vi "Fct_Direction_vent.vi"(11 "Tension Girouette":dbl) -> (3 "Chaîne":string)   [LabVIEW 2017]
doc: "Ce VI donne à partir d'une tension d'entrée, les point cardinaux.\n\nCopyright | Jixiong Liu & Benoit Mangeard"
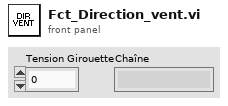
[diagram p1: front panel]
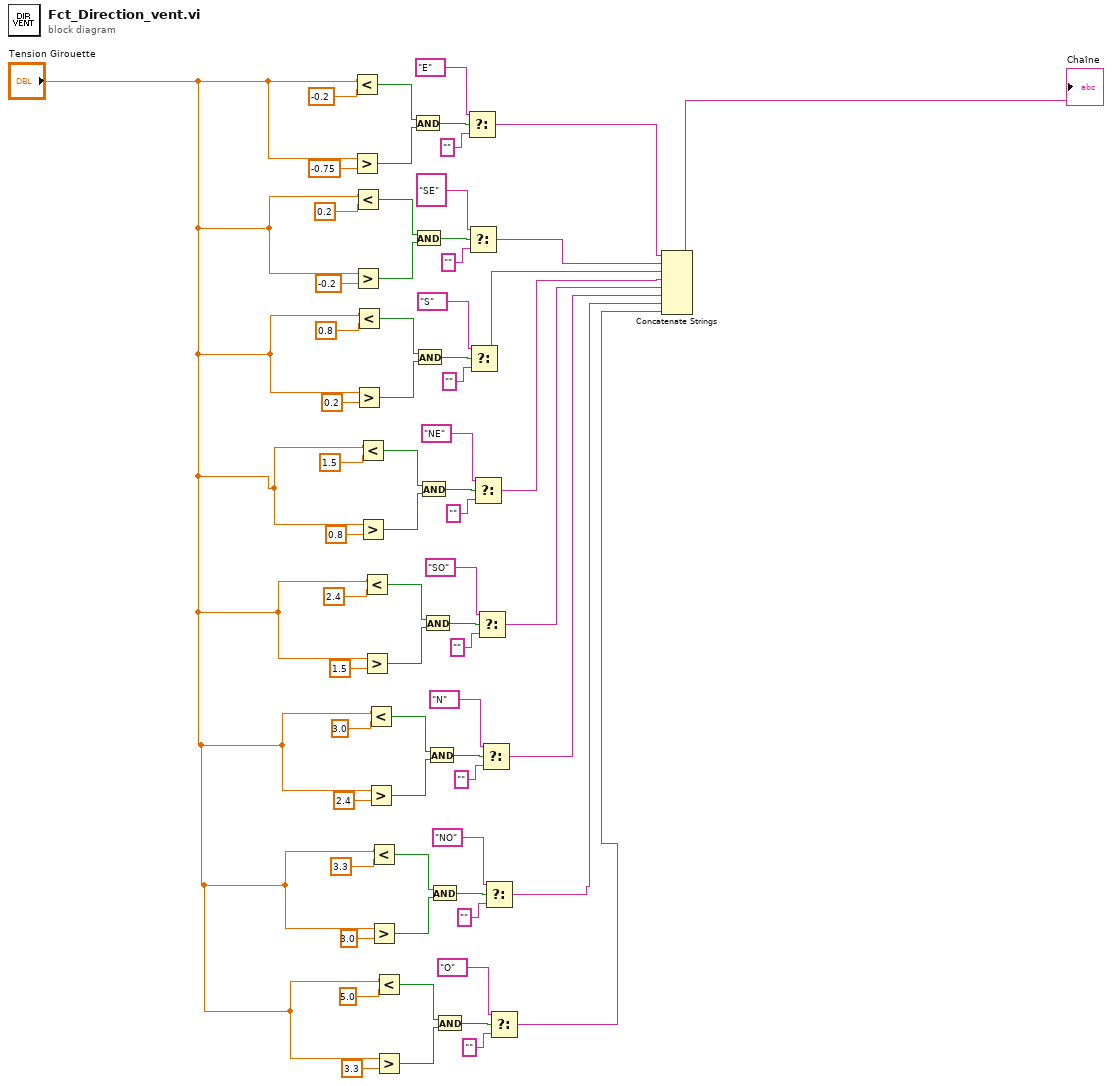
[diagram p0: block diagram]
diagram:
  n1 = Less?(x="Tension Girouette", y=-0.2) -> (x < y?=w64:bool)
  n2 = Greater?(x="Tension Girouette", y=-0.75) -> (0:w63:bool)
  n3 = Less?(x="Tension Girouette", y=0.2) -> (x < y?=w56:bool)
  n4 = Greater?(x="Tension Girouette", y=-0.2) -> (0:w55:bool)
  n5 = Less?(x="Tension Girouette", y=0.8) -> (x < y?=w49:bool)
  n6 = Greater?(x="Tension Girouette", y=0.2) -> (0:w48:bool)
  n7 = Less?(x="Tension Girouette", y=1.5) -> (x < y?=w42:bool)
  n8 = Greater?(x="Tension Girouette", y=0.8) -> (0:w41:bool)
  n9 = Less?(x="Tension Girouette", y=2.4) -> (x < y?=w35:bool)
  n10 = Greater?(x="Tension Girouette", y=1.5) -> (0:w34:bool)
  n11 = Less?(x="Tension Girouette", y=3.0) -> (x < y?=w28:bool)
  n12 = Greater?(x="Tension Girouette", y=2.4) -> (0:w27:bool)
  n13 = Less?(x="Tension Girouette", y=3.3) -> (x < y?=w21:bool)
  n14 = Greater?(x="Tension Girouette", y=3.0) -> (0:w20:bool)
  n15 = Less?(x="Tension Girouette", y=5.0) -> (x < y?=w14:bool)
  n16 = Greater?(x="Tension Girouette", y=3.3) -> (0:w13:bool)
  n17 = And(x=w64, y=w63) -> (x .and. y?=w62:bool)
  n18 = And(x=w56, y=w55) -> (x .and. y?=w54:bool)
  n19 = And(x=w49, y=w48) -> (x .and. y?=w47:bool)
  n20 = And(x=w42, y=w41) -> (x .and. y?=w40:bool)
  n21 = And(x=w35, y=w34) -> (x .and. y?=w33:bool)
  n22 = And(x=w28, y=w27) -> (x .and. y?=w26:bool)
  n23 = And(x=w21, y=w20) -> (x .and. y?=w19:bool)
  n24 = And(x=w14, y=w13) -> (x .and. y?=w12:bool)
  n25 = Select(t="E", s=w62, f="" ("cas faux")) -> (s? t:f=w8:string)
  n26 = Select(t="SE", s=w54, f="" ("cas faux")) -> (s? t:f=w7:string)
  n27 = Select(t="S", s=w47, f="" ("cas faux")) -> (s? t:f=w6:string)
  n28 = Select(t="NE", s=w40, f="" ("cas faux")) -> (s? t:f=w5:string)
  n29 = Select(t="SO", s=w33, f="" ("cas faux")) -> (s? t:f=w4:string)
  n30 = Select(t="N", s=w26, f="" ("cas faux")) -> (s? t:f=w3:string)
  n31 = Select(t="NO", s=w19, f="" ("cas faux")) -> (s? t:f=w2:string)
  n32 = Select(t="O", s=w12, f="" ("cas faux")) -> (s? t:f=w1:string)
  n33 = Concatenate Strings(w8, w7, w6, w5, w4, w3, w2, w1) -> (→"Chaîne":string)
